vi "Read 1 Key Tap.vi"(8 "Error In":errorcluster, 11 "Leap Handle":T6) -> (0 "Error Out":errorcluster, 1 "Key Tap Status":T1, 2 "Key Tap":T2={"Common"={"ID"=0.0, "Duration (S)"=0.0, "Gesture Type"=enum."Invalid", "Gesture State"=enum."Invalid"}, "Direction"={"Pitch"=nan, "Yaw"=nan, "Roll"=nan, "Magnitude"=nan, "XYZ"=[nan, nan, nan]}, "Position"={"Pitch"=nan, "Yaw"=nan, "Roll"=nan, "Magnitude"=nan, "XYZ"=[nan, nan, nan]}, "Progress"=0.0}, 3 "Leap Handle":T6)   [LabVIEW 2014, in "LMH-Leap.lvlib"]
doc: "Read all data from one key tap gesture."
uses:
  LMH-Leap.lvlib
  Private/Type Defs/Leap Handle.ctl
  C:/github/makerhub/Leap/LabVIEW/vi.lib/LabVIEW Hacker/Leap/Private/Libs/LeapCSharp.NET3.5.dll
  LabVIEW Hacker/Leap/Private/Libs/LeapCSharp.NET3.5.dll
  Private/Type Defs/Gesture Key Tap.ctl
  Private/Type Defs/Gesture Common.ctl
  Private/Type Defs/Gesture Type.ctl
  Private/Type Defs/Gesture State.ctl
  Private/Type Defs/Vector.ctl
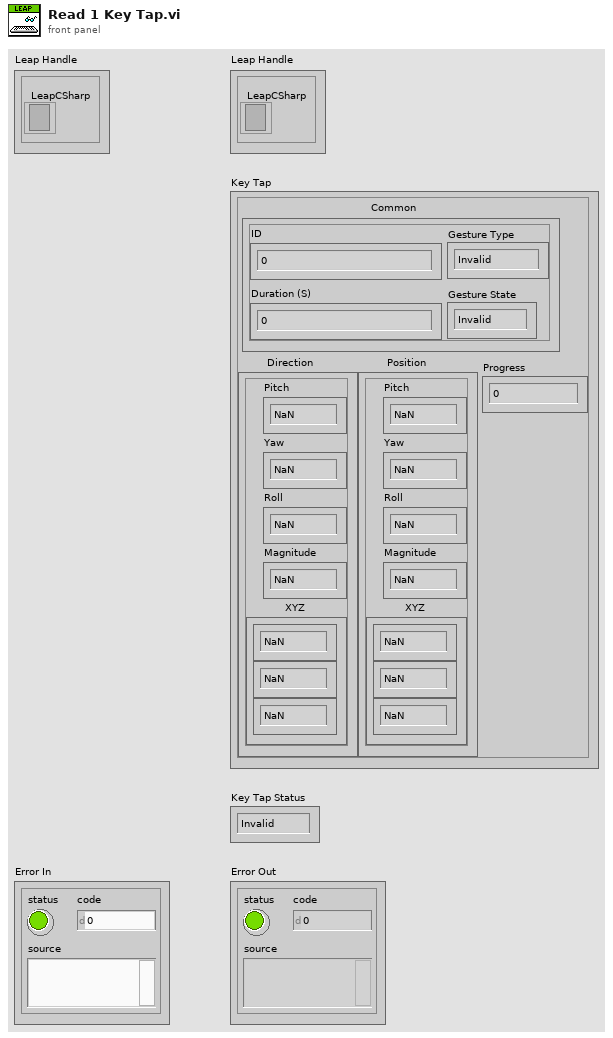
[diagram p1: front panel]
types:
  T1 = typedef "LMH-Leap.lvlib/Gesture State.ctl" = enum16{"Invalid", "Start", "Update", "Stop"}
  T2 = typedef "LMH-Leap.lvlib/Gesture Key Tap.ctl" = cluster{"Common":T3, "Direction":T5, "Position":T5, "Progress":dbl}
  T3 = typedef "LMH-Leap.lvlib/Gesture Common.ctl" = cluster{"ID":dbl, "Duration (S)":dbl, "Gesture Type":T4, "Gesture State":T1}
  T4 = typedef "LMH-Leap.lvlib/Gesture Type.ctl" = enum16{"Invalid", "Swipe", "Circle", "Screen Tap", "Key Tap"}
  T5 = typedef "LMH-Leap.lvlib/Vector.ctl" = cluster{"Pitch":sgl, "Yaw":sgl, "Roll":sgl, "Magnitude":sgl, "XYZ":sgl[]}
  T6 = typedef "LMH-Leap.lvlib/Leap Handle.ctl" = cluster{"LeapCSharp":refnum<k24>}
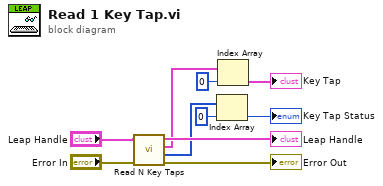
[diagram p0: block diagram]
diagram:
  n1 = call "Read N Key Taps.vi"("Error In"="Error In", "Leap Handle"="Leap Handle") -> ("Error Out"=→"Error Out":errorcluster, "Key Tap Statuses"=w2:T1[], "Key Tap Gestures"=w4:T2[], "Leap Handle"=→"Leap Handle":T6)  [unwired: 6 in]
  n2 = Index Array(array=w2, index=0) -> (element=→"Key Tap Status":T1)
  n3 = Index Array(array=w4, index=0) -> (element=→"Key Tap":T2)
